vi "相机2-计算螺杆末端在P10时位置信息.vi"(9 "拍螺杆功能选择":T2=enum."换刀或者换夹持机构后计算螺杆末端偏移量P10拍照", 11 "Image in":T3) -> (0 "校准2：换刀或夹持机构后螺杆末端位置变化量":T1 {"X" format="%#.3f"}, 3 "Img out":T3(plugin-control))   [LabVIEW 2014]
uses:
  Global.vi
  Controls/XYPos.ctl
  <vilib>/vision/Measure.llb/Edge Polarity.ctl
  <vilib>/vision/Measure.llb/Edge Options.ctl
  <vilib>/vision/Image Controls.llb/IMAQ Image.ctl
panel:
  in  "Img Path":path=path "D:/测试图片/20200714/771自动锁螺丝/NG图片-相机1/771自动锁螺丝_NG图片-相机1_20200714-085746.jpg"
  # "-180 顺时针为正  参考影像坐标系统"
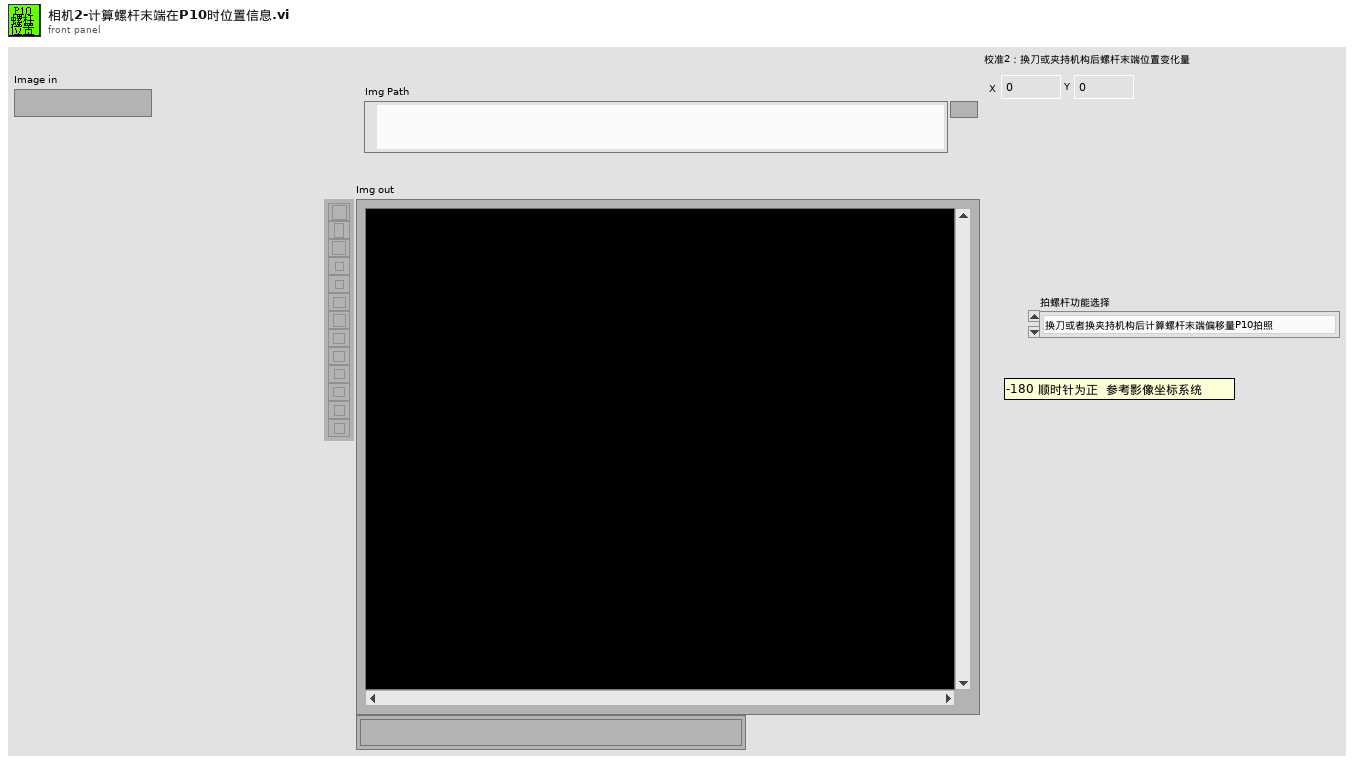
[diagram p1: front panel]
types:
  T1 = typedef "XYPos.ctl" = cluster{"X":dbl, "Y":dbl}
  T2 = typedef "控件-拍照螺杆末端功能选择.ctl" = enum16{"第一次螺杆对孔完成后记录螺杆末端图像P10拍照", "换刀或者换夹持机构后计算螺杆末端偏移量P10拍照"}
  T3 = typedef "IMAQ Image.ctl" = refnum<image>
  T4 = typedef "Edge Options.ctl" = cluster{"Edge Polarity":T5, "Kernel Size":u32, "Width":u32, "Minimum Edge Strength":sgl, "Interpolation Type":enum32{"Zero Order", "Bilinear", "Quadratic", "Cubic", "Bilinear Fixed"}, "Data Processing Method":enum32{"Average", "Median"}}
  T5 = typedef "Edge Polarity.ctl" = u32
  T6 = cluster{"Search  Direction":u32, "Edge Options":T4, "Show Search Area":bool, "Show Search Lines":bool, "Show Edges Found":bool, "Show Result":bool, "Search Area Color":u32, "Search Lines Color":u32, "Edge Locations Color":u32, "Result Color":u32, "Overlay Group Name":string}
  T7 = cluster{"Center (Pixels)":cluster{"X":sgl, "Y":sgl}, "Radius (Pixels)":dbl, "Center (Real-World)":cluster{"X":sgl, "Y":sgl}, "Radius (Real-World)":dbl, "Roundness (Real-World)":dbl, "Average Strength":dbl, "Average SNR (dB)":dbl}
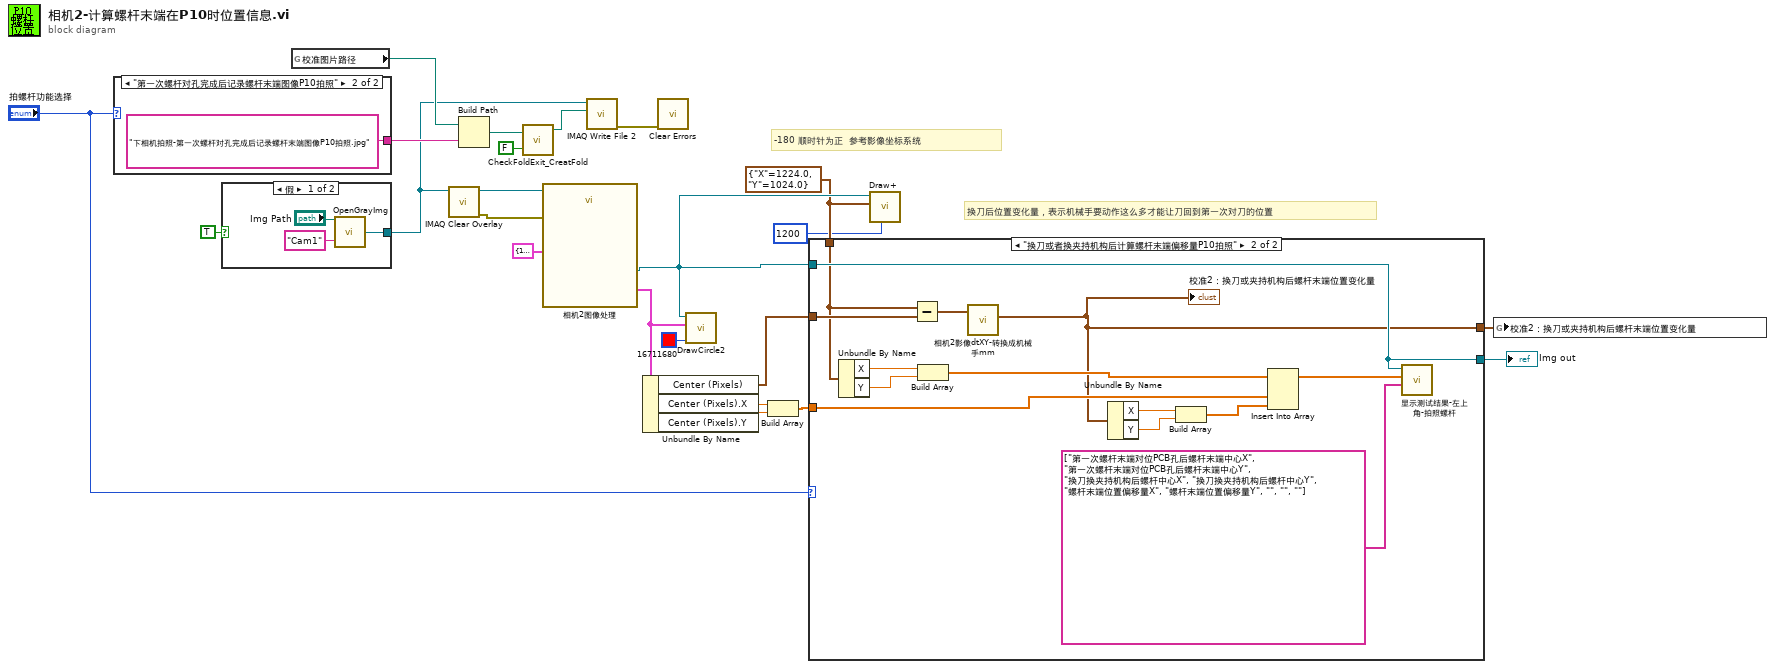
[diagram p0: block diagram]
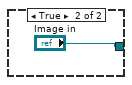
[diagram p2: hidden frame]
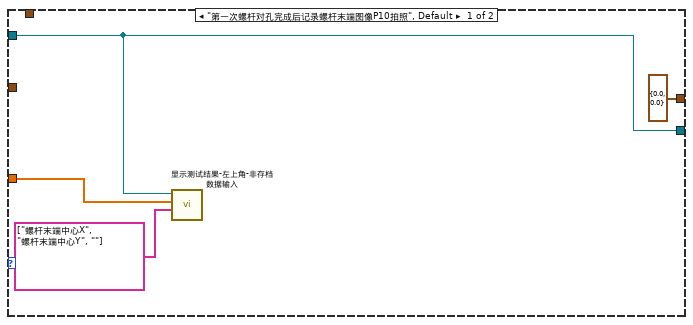
[diagram p3: hidden frame]
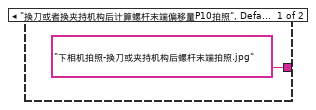
[diagram p4: hidden frame]
diagram:
  w2 = T1 {"X"=1224.0, "Y"=1024.0} ("坐标")
  # "-180 顺时针为正  参考影像坐标系统"
  # "换刀后位置变化量，表示机械手要动作这么多才能让刀回到第一次对刀的位置"
  n1 = case shown="\"第一次螺杆对孔完成后记录螺杆末端图像P10拍照\"" "拍螺杆功能选择" {
    tunnel: ["下相机拍照-换刀或夹持机构后螺杆末端拍照.jpg" ("time format string (%c)") "下相机拍照-第一次螺杆对孔完成后记录螺杆末端图像P10拍照.jpg" ("time format string (%c)")] -> w15
    frame "换刀或者换夹持机构后计算螺杆末端偏移量P10拍照", Default {
    }
    frame "第一次螺杆对孔完成后记录螺杆末端图像P10拍照" {
    }
  }
  n2 = case shown="假" TRUE {
    tunnel: [w27 "Image in"] -> w9
    frame False {
      n3 = call "OpenGrayImg.vi"("Image Name"="Cam1", "Img Path"="Img Path") -> ("Image Out"=w27:T3)
    }
    frame True {
    }
  }
  n4 = global read "Global.vi" "校准图片路径"() -> (w21:path)
  n5 = call "IMAQ Clear Overlay"("Image"=w9) -> ("error out"=w22:errorcluster, "Image Out"=w23:T3)  [unwired: 9 in]
  n6 = Build Path(base path=w21, name or relative path=w15) -> (appended path=w19:path)
  n7 = call "CheckFoldExit_CreatFold.vi"("path in"=w19, "FoldOrFile¡H"=FALSE) -> ("File out"=w17:path)  [unwired: 2 out]
  n8 = call "相机2图像处理"("Image In"=w23, "Options (螺杆末端)"=T6 {"Search  Direction"=1, "Edge Options"={"Edge Polarity"=2, "Kernel Size"=11, "Width"=11, "Minimum Edge Strength"=40.0, "Interpolation Type"=enum."Bilinear Fixed", "Data Processing Method"=enum."Average"}, "Show Search Area"=FALSE, "Show Search Lines"=FALSE, "Show Edges Found"=TRUE, "Show Result"=FALSE, "Search Area Color"=65280, "Search Lines Color"=255, "Edge Locations Color"=16776960, "Result Color"=16711680, "Overlay Group Name"=""}, "error in"=w22) -> ("Image Out"=w5:T3, "Fitted Circle (螺杆末端)"=w4:T7)  [unwired: 22 in, 1 out]
  n9 = call-poly "IMAQ Write File 2"("File Path"=w17, "Image"=w9) -> ("error out"=w20:errorcluster)  [unwired: 8 in, 1 out]
  n10 = Unbundle By Name(w4) -> ("Center (Pixels)"=w6:cluster{"X":sgl, "Y":sgl}, "Center (Pixels).X"=w14:sgl, "Center (Pixels).Y"=w13:sgl)
  n11 = call <vilib>:"Clear Errors.vi"("error in (no error)"=w20) -> ()  [unwired: 5 in, 2 out]
  n12 = call "DrawCircle2.vi"("Color"=u32 16711680, "Fitted Circle (左圆)"=w4, "Img in"=w5) -> ()  [unwired: 1 in, 1 out]
  n13 = Build Array(w14, w13) -> (w16:sgl[])
  n14 = case shown="\"换刀或者换夹持机构后计算螺杆末端偏移量P10拍照\"" "拍螺杆功能选择" {
    tunnel: w5 -> [w31 w43]
    tunnel: w16 -> [w33 w38]
    tunnel: w6 -> [_ w47]
    tunnel: [w31 w43] -> w11
    tunnel: w2 -> [_ w35]
    tunnel: [T1 {"X"=0.0, "Y"=0.0} ("机械手移动量 mm") w34] -> w8
    frame "第一次螺杆对孔完成后记录螺杆末端图像P10拍照", Default {
      n15 = call "显示测试结果-左上角-非存档数据输入.vi"("量测项目名称"=string[] ["螺杆末端中心X", "螺杆末端中心Y", ""], "显示数据"=w33, "Img输入"=w31) -> ()  [unwired: 8 in, 1 out]
    }
    frame "换刀或者换夹持机构后计算螺杆末端偏移量P10拍照" {
      n16 = Unbundle By Name(w35) -> ("X"=w45:dbl, "Y"=w44:dbl)
      n17 = Subtract(x=w35, y=w47) -> (x-y=w42:T1)
      n18 = Build Array(w45, w44) -> (w39:dbl[])
      n19 = call "相机2影像dtXY-转换成机械手mm.vi"("相机2影像偏移量"=w42) -> ("机械手移动量 mm"=w34:T1)  [unwired: 10 in]
      "校准2：换刀或夹持机构后螺杆末端位置变化量" <- w34
      n20 = Unbundle By Name(w34) -> ("X"=w40:dbl, "Y"=w41:dbl)
      n21 = Build Array(w40, w41) -> (w36:dbl[])
      n22 = Insert Into Array(array=w39, new element #1=w38, new element #2=w36) -> (w37:dbl[])  [unwired: 1 in]
      n23 = call "显示测试结果-左上角-拍照螺杆.vi"("量测项目名称"=string[] ["第一次螺杆末端对位PCB孔后螺杆末端中心X", "第一次螺杆末端对位PCB孔后螺杆末端中心Y", "换刀换夹持机构后螺杆中心X", "换刀换夹持机构后螺杆中心Y", "螺杆末端位置偏移量X", "螺杆末端位置偏移量Y", "", "", ""], "显示数据"=w37, "Img输入"=w43) -> ()  [unwired: 9 in]
    }
  }
  "Img out" <- w11
  n24 = call "Draw+.vi"("Width"=1200, "input cluster"=w2, "Image In"=w5) -> ()  [unwired: 3 in, 1 out]
  n25 = global write "Global.vi" "校准2：换刀或夹持机构后螺杆末端位置变化量"(w8) -> ()
